vi "1.vi"(8 "error in (no error)":errorcluster, 11 "Array":dbl[][](array[numeric])) -> (0 "error in (no error) (dup)":errorcluster, 3 "identify matrix?":bool)   [LabVIEW 2017]
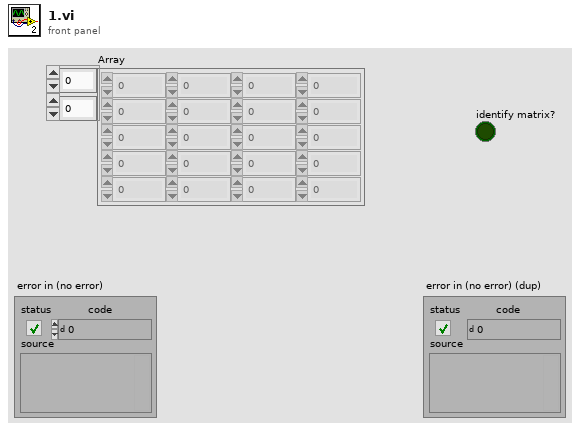
[diagram p1: front panel]
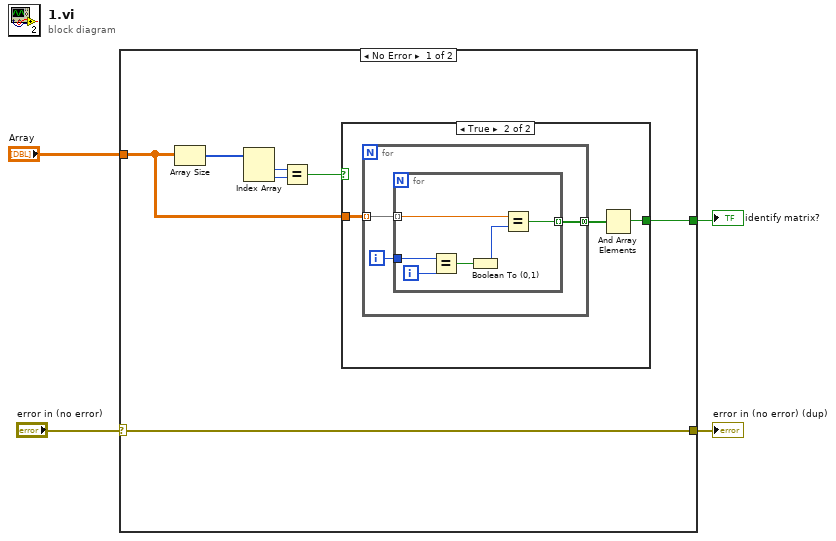
[diagram p0: block diagram]
diagram:
  n1 = case shown="No Error" "error in (no error)" {
    selector: "error in (no error)" -> [w5 w24]
    tunnel: "Array" -> [w8 _]
    tunnel: [w6 _] -> w3
    tunnel: [w5 w24] -> w1
    frame No Error {
      n2 = Array Size(array=w8) -> (size(s)=w11:i32[])
      n3 = Index Array(array=w11) -> (element #1=w10:i32, element #2=w9:i32)  [unwired: 2 in]
      n4 = Equal?(x=w10, y=w9) -> (x = y?=w7:bool)
      n5 = case shown="True" w7 {
        tunnel: w8 -> [_ w14]
        tunnel: [_ w12] -> w6
        frame False {
        }
        frame True {
          n6 = for {
            tunnel: w14 -> [w16] mode=indexing
            tunnel: [w15] -> w13 mode=concatenating
            i -> [w17]
            n7 = for {
              tunnel: w17 -> [w23]
              tunnel: w16 -> [w20] mode=indexing
              tunnel: [w18] -> w15 mode=indexing
              i -> [w22]
              n8 = Equal?(x=w23, y=w22) -> (x = y?=w21:bool)
              n9 = Boolean To (0,1)(Boolean=w21) -> (0, 1=w19:i16)
              n10 = Equal?(x=w20, y=w19) -> (x = y?=w18:bool)
            }
          }
          n11 = And Array Elements(Boolean array=w13) -> (logical AND=w12:bool)
        }
      }
    }
    frame Error {
    }
  }
  "identify matrix?" <- w3
  "error in (no error) (dup)" <- w1
